vi "Receive I32 Value Msg.vi"(8 "error in (no error)":errorcluster, 10 "I32ValueMsg":refnum<class "I32ValueMsg.lvclass">, 11 "TopLevelApplication in":refnum<class "TopLevelApplication.lvclass">) -> (0 "error out":errorcluster, 3 "TopLevelApplication out":refnum<class "TopLevelApplication.lvclass">)   [LabVIEW 2015, in "TopLevelApplication.lvlib" / "TopLevelApplication.lvclass"]
uses:
  TopLevelApplication.lvclass
  AutoRegistration/ActorAutoRegistration Messages/I32ValueMsg/I32ValueMsg.lvclass
  Dialog Box Implementations/OneButtonDialogBox/OneButtonDialogBox.lvclass
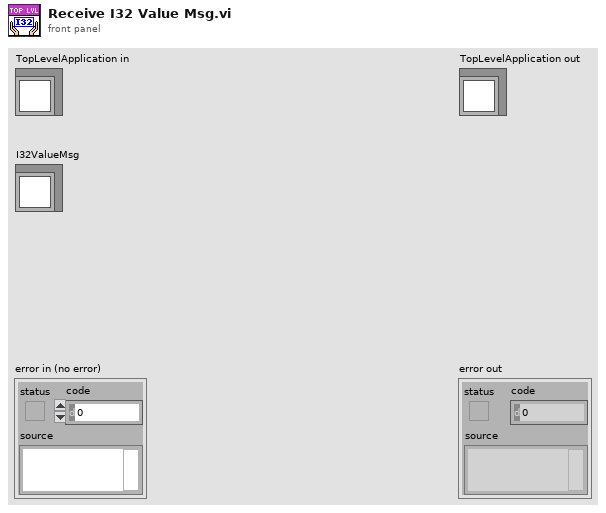
[diagram p1: front panel]
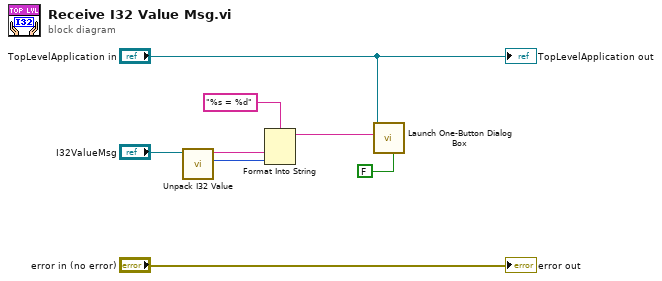
[diagram p0: block diagram]
diagram:
  n1 = call-dynamic "Unpack I32 Value.vi"("I32ValueMsg in"="I32ValueMsg") -> ("Value"=w5:i32, "Name"=w6:string)  [unwired: 9 in]
  n2 = Format Into String(format string="%s = %d", w6, w5) -> (resulting string=w2:string)  [unwired: 2 in, 1 out]
  n3 = call "Launch One-Button Dialog Box.vi"("Modal? (T)"=FALSE, "Message Text"=w2, "Dialog Launcher"="TopLevelApplication in") -> ()  [unwired: 8 in, 1 out]
  "error out" <- "error in (no error)"
  "TopLevelApplication out" <- "TopLevelApplication in"
